vi "Global.vi"() -> ()   [LabVIEW 2013]
panel:
  in  "Regler aktiv":bool
  in  "Wegzähler":dbl
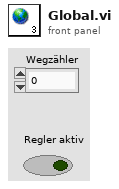
[diagram p1: front panel]
diagram:
